vi "Move.vi"(7 "Part 1":bool, 8 "error in (no error)":errorcluster, 11 "Burrow in":refnum<class "Burrow.lvclass">) -> (0 "error out":errorcluster)   [LabVIEW 2019, in "23.lvlib" / "Burrow.lvclass"]
uses:
  Burrow.lvclass
  Amphipod/Amphipod.lvclass
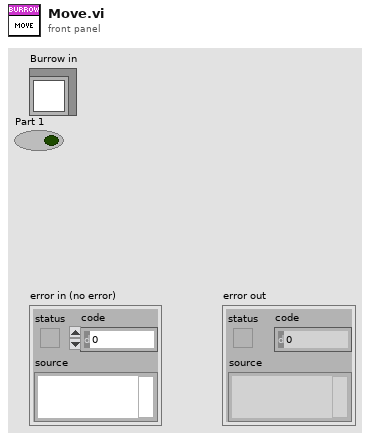
[diagram p1: front panel]
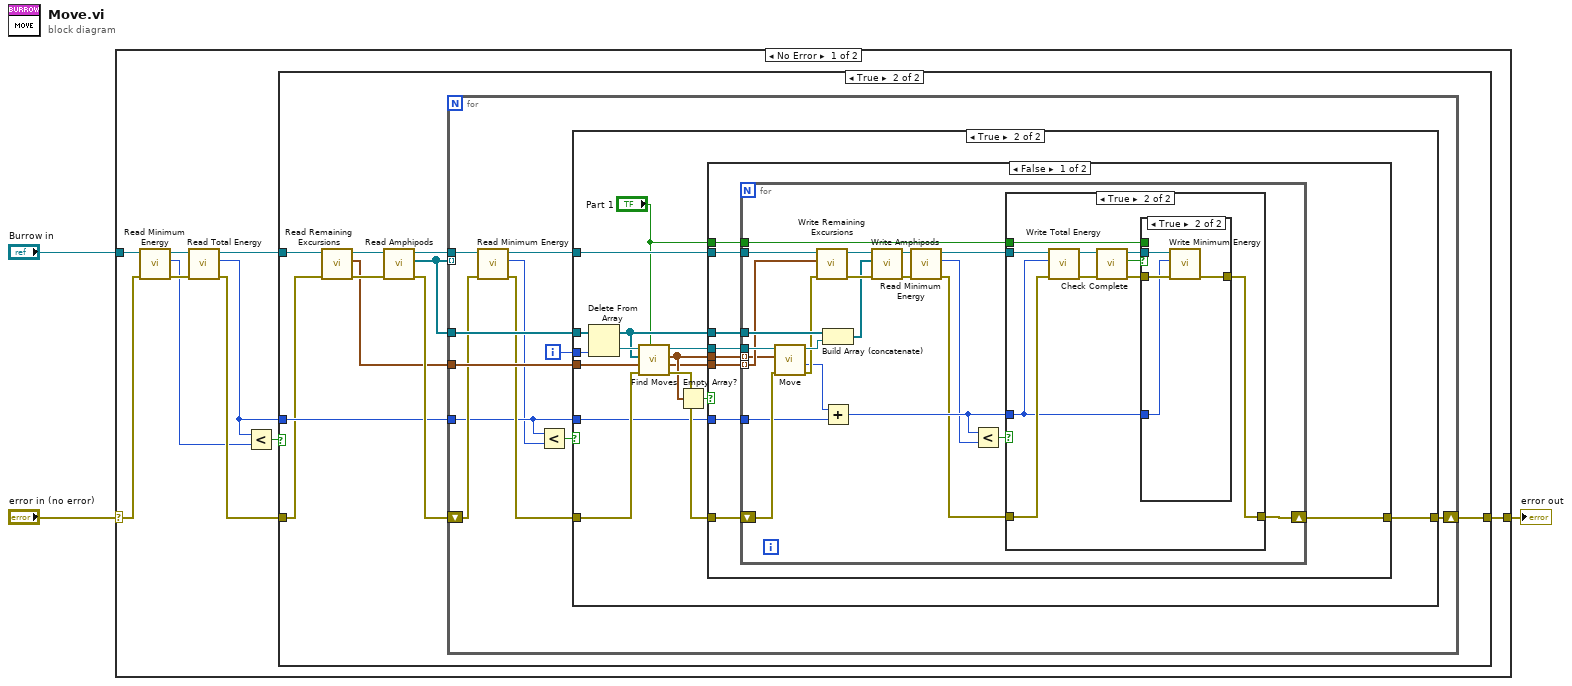
[diagram p0: block diagram]
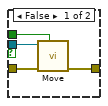
[diagram p5: hidden frame]
diagram:
  n1 = case shown="No Error" "error in (no error)" {
    selector: "error in (no error)" -> [w8 w103]
    tunnel: [w11 w103] -> w2
    tunnel: "Burrow in" -> [w9 _]
    frame No Error {
      n2 = call-dynamic "Read Minimum Energy.vi"("error in (no error)"=w8, "Burrow in"=w9) -> ("error out"=w7:errorcluster, "Minimum Energy"=w4:u64, "Burrow out"=w10:refnum<class "Burrow.lvclass">)  [unwired: 7 in]
      n3 = call-dynamic "Read Total Energy.vi"("error in (no error)"=w7, "Burrow in"=w10) -> ("error out"=w12:errorcluster, "Total Energy"=w6:u64, "Burrow out"=w13:refnum<class "Burrow.lvclass">)  [unwired: 7 in]
      n4 = Less?(x=w6, y=w4) -> (x < y?=w5:bool)
      n5 = case shown="True" w5 {
        tunnel: w13 -> [_ w18]
        tunnel: w12 -> [w14 w16]
        tunnel: [w14 w22] -> w11
        tunnel: w6 -> [_ w20]
        frame False {
        }
        frame True {
          n6 = call-dynamic "Read Remaining Excursions.vi"("error in (no error)"=w16, "Burrow in"=w18) -> ("error out"=w17:errorcluster, "Remaining Excursions"=w15:cluster{"A":u8, "B":u8, "C":u8, "D":u8}, "Burrow out"=w19:refnum<class "Burrow.lvclass">)  [unwired: 7 in]
          n7 = call-dynamic "Read Amphipods.vi"("error in (no error)"=w17, "Burrow in"=w19) -> ("error out"=w24:errorcluster, "Amphipods"=w23:refnum<class "Amphipod.lvclass">[], "Burrow out"=w21:refnum<class "Burrow.lvclass">)  [unwired: 7 in]
          n8 = for {
            tunnel: w21 -> [w30]
            tunnel: w23 -> [_] mode=indexing
            tunnel: w20 -> [w27]
            tunnel: w23 -> [w35]
            shift-right: [w34] -> w22
            shift-left: w24 -> [w29]
            tunnel: w15 -> [w32]
            i -> [w33]
            n9 = call-dynamic "Read Minimum Energy.vi"("error in (no error)"=w29, "Burrow in"=w30) -> ("error out"=w28:errorcluster, "Minimum Energy"=w26:u64, "Burrow out"=w31:refnum<class "Burrow.lvclass">)  [unwired: 7 in]
            n10 = Less?(x=w27, y=w26) -> (x < y?=w25:bool)
            n11 = case shown="True" w25 {
              tunnel: w35 -> [_ w51]
              tunnel: [w36 w50] -> w34
              tunnel: w33 -> [_ w49]
              tunnel: w32 -> [_ w42]
              tunnel: w31 -> [_ w40]
              tunnel: w28 -> [w36 w39]
              tunnel: w27 -> [_ w38]
              frame False {
              }
              frame True {
                n12 = Delete From Array(array=w51, index=w49) -> (deleted portion=w48:refnum<class "Amphipod.lvclass">, array with subset deleted=w47:refnum<class "Amphipod.lvclass">[])  [unwired: 1 in]
                n13 = call-dynamic "Find Moves.vi"("Part 1"="Part 1", "error in (no error)"=w39, "Remaining Excursions"=w42, "Amphipods in"=w47, "Amphipod in"=w48) -> ("error out"=w46:errorcluster, "Remaining Excursions for Moves"=w41:cluster{"A":u8, "B":u8, "C":u8, "D":u8}[], "Valid Moves"=w44:cluster{"Row":i8, "Column":i8}[], "Amphipod out"=w45:refnum<class "Amphipod.lvclass">)  [unwired: 3 in]
                n14 = Empty Array?(array=w44) -> (empty?=w43:bool)
                n15 = case shown="False" w43 {
                  tunnel: w40 -> [w60 _]
                  tunnel: w38 -> [w59 _]
                  tunnel: [w58 w102] -> w50
                  tunnel: w47 -> [w57 _]
                  tunnel: w46 -> [w56 w102]
                  tunnel: w45 -> [w55 _]
                  tunnel: w44 -> [w54 _]
                  tunnel: w41 -> [w53 _]
                  tunnel: "Part 1" -> [w52 _]
                  frame False {
                    n16 = for {
                      tunnel: w60 -> [w74]
                      tunnel: w54 -> [w65] mode=indexing
                      tunnel: w59 -> [w64]
                      shift-right: [w78] -> w58
                      shift-left: w56 -> [w79]
                      tunnel: w57 -> [w80]
                      tunnel: w55 -> [w82]
                      tunnel: w53 -> [w73] mode=indexing
                      tunnel: w52 -> [w61]
                      n17 = call-dynamic "Move.vi"("error in (no error)"=w79, "New Position"=w65, "Amphipod in"=w82) -> ("error out"=w72:errorcluster, "Energy Used"=w63:u64, "Amphipod out"=w81:refnum<class "Amphipod.lvclass">)  [unwired: 5 in, 1 out]
                      n18 = call-dynamic "Write Remaining Excursions.vi"("error in (no error)"=w72, "Remaining Excursions"=w73, "Burrow in"=w74) -> ("error out"=w71:errorcluster, "Burrow out"=w75:refnum<class "Burrow.lvclass">)  [unwired: 7 in]
                      n19 = Build Array (concatenate)(w80, w81) -> (w62:refnum<class "Amphipod.lvclass">[])
                      n20 = Add(x=w63, y=w64) -> (x+y=w77:u64)
                      n21 = call-dynamic "Write Amphipods.vi"("error in (no error)"=w71, "Amphipods"=w62, "Burrow in"=w75) -> ("error out"=w68:errorcluster, "Burrow out"=w70:refnum<class "Burrow.lvclass">)  [unwired: 7 in]
                      n22 = call-dynamic "Read Minimum Energy.vi"("error in (no error)"=w68, "Burrow in"=w70) -> ("error out"=w67:errorcluster, "Minimum Energy"=w66:u64, "Burrow out"=w69:refnum<class "Burrow.lvclass">)  [unwired: 7 in]
                      n23 = Less?(x=w77, y=w66) -> (x < y?=w76:bool)
                      n24 = case shown="True" w76 {
                        tunnel: w69 -> [_ w87]
                        tunnel: w67 -> [w83 w86]
                        tunnel: [w83 w88] -> w78
                        tunnel: w77 -> [_ w85]
                        tunnel: w61 -> [_ w84]
                        frame False {
                        }
                        frame True {
                          n25 = call-dynamic "Write Total Energy.vi"("error in (no error)"=w86, "Score"=w85, "Burrow in"=w87) -> ("error out"=w92:errorcluster, "Burrow out"=w93:refnum<class "Burrow.lvclass">)  [unwired: 7 in]
                          n26 = call-dynamic "Check Complete.vi"("error in (no error)"=w92, "Burrow in"=w93) -> ("error out"=w91:errorcluster, "Complete?"=w89:bool, "Burrow out"=w90:refnum<class "Burrow.lvclass">)  [unwired: 7 in]
                          n27 = case shown="True" w89 {
                            tunnel: w91 -> [w97 w100]
                            tunnel: w90 -> [w96 w101]
                            tunnel: w85 -> [_ w99]
                            tunnel: [w95 w98] -> w88
                            tunnel: w84 -> [w94 _]
                            frame False {
                              n28 = call-dynamic "Move.vi"("Part 1"=w94, "error in (no error)"=w97, "Burrow in"=w96) -> ("error out"=w95:errorcluster)  [unwired: 8 in]
                            }
                            frame True {
                              n29 = call-dynamic "Write Minimum Energy.vi"("error in (no error)"=w100, "Minimum Energy"=w99, "Burrow in"=w101) -> ("error out"=w98:errorcluster)  [unwired: 7 in, 1 out]
                            }
                          }
                        }
                      }
                    }
                  }
                  frame True {
                  }
                }
              }
            }
          }
        }
      }
    }
    frame Error {
    }
  }
  "error out" <- w2
